vi "file_path.vi"() -> (0 "cancelled":bool, 3 "selected path":path)   [LabVIEW 2011]
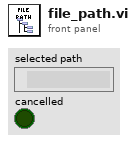
[diagram p1: front panel]
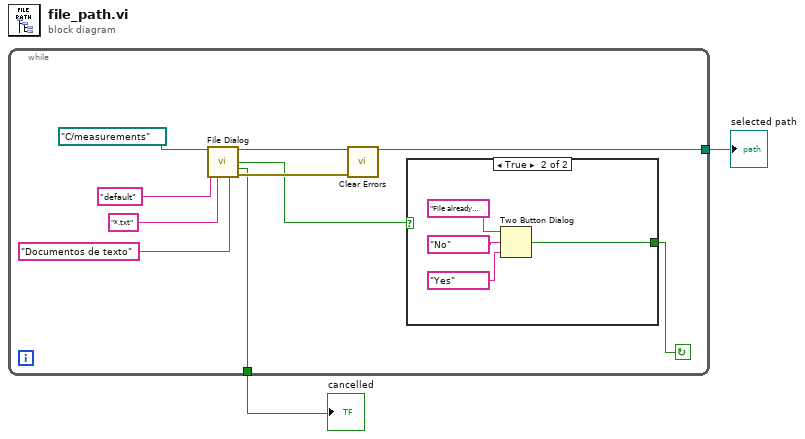
[diagram p0: block diagram]
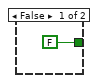
[diagram p2: hidden frame]
diagram:
  n1 = while {
    tunnel: [w5] -> w2
    tunnel: [w3] -> w1
    stop <- w4 continue-if-true
    n2 = call "File Dialog"("start path"=path "C:/measurements", "default name"="default", "pattern (all files)"="*.txt", "pattern label"="Documentos de texto") -> ("selected path"=w5:path, "exists"=w7:bool, "cancelled"=w3:bool, "error out"=w11:errorcluster)  [unwired: 8 in]
    n3 = call <vilib>:"Clear Errors.vi"("error in (no error)"=w11) -> ()  [unwired: 6 in, 1 out]
    n4 = case shown="True" w7 {
      tunnel: [FALSE ("T button?") w13] -> w4
      frame False {
      }
      frame True {
        n5 = Two Button Dialog(message="File already exits. Do you want to replace it?", 1:"Yes" ("message"), 2:"No" ("message")) -> (T button?=w13:bool)
      }
    }
  }
  "selected path" <- w2
  "cancelled" <- w1
